vi "niRFUtil WFM Replace Waveform Segment (real wfm).vi"(4 "Waveform Segment":T2 {"y" min=0 max=127 format="%.2f"; "dx" format="%^.2e"; "x0" format="%^.2e"}, 5 "WFM replace mode":T1, 6 "Default Value (0)":sgl min=0 max=127 format="%.2f", 7 "Waveform In":T2 {"y" min=0 max=127 format="%.2f"; "dx" format="%^.2e"; "x0" format="%^.2e"}) -> (3 "Waveform Out":T2 {"y" min=0 max=127 format="%.2f"; "dx" format="%^.2e"; "x0" format="%^.2e"})   [LabVIEW 2015, in "niRFUtil.lvlib"]
doc: "(c) Copyright 2006, National Instruments, Inc. This VI may not be duplicated, sold, or distributed without written consent from National Instruments."
uses:
  niRFUtil.lvlib
  Includes/niRFUtil INC Real Waveform.ctl
  Includes/niRFUtil INC Real Array.ctl
  Includes/niRFUtil INC Waveform Replace Mode.ctl
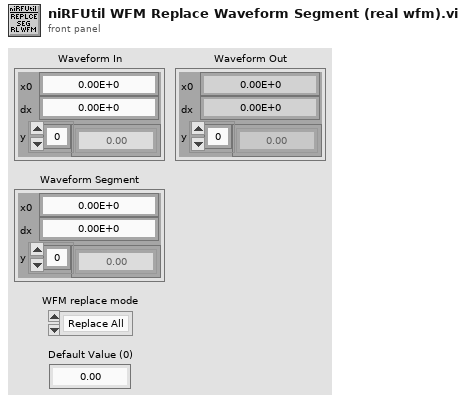
[diagram p1: front panel]
types:
  T1 = typedef "niRFUtil.lvlib/niRFUtil INC Waveform Replace Mode.ctl" = enum16{"Replace All", "Replace Pt By Pt"}
  T2 = typedef "niRFUtil.lvlib/niRFUtil INC Real Waveform.ctl" = cluster{"x0":dbl, "dx":dbl, "y":T3}
  T3 = typedef "niRFUtil.lvlib/niRFUtil INC Real Array.ctl" = sgl[]
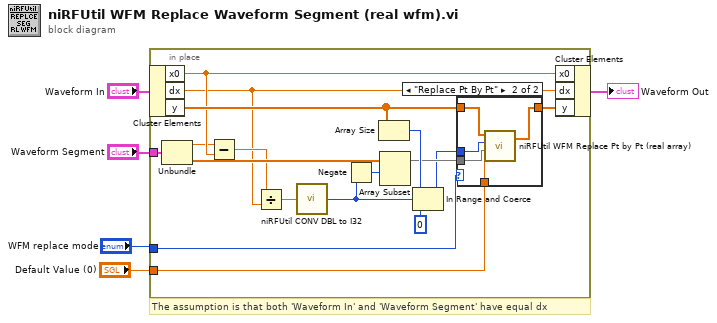
[diagram p0: block diagram]
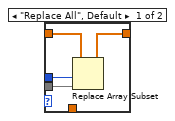
[diagram p2: hidden frame]
diagram:
  # "The assumption is that both 'Waveform In' and 'Waveform Segment' have equal dx"
  n1 = in-place {
    in-place-border: "Waveform Segment" -> [w22]
    in-place-border: "WFM replace mode" -> [w13]
    in-place-border: "Default Value (0)" -> [w12]
    n2 = in-place-cluster #1("Waveform In") -> ("x0"=w9:dbl, "dx"=w7:dbl, "y"=w15:T3)
    n3 = Unbundle(w22) -> ("x0"=w8:dbl, "y"=w19:T3)  [unwired: 1 out]
    n4 = Subtract(x=w8, y=w9) -> (x-y=w11:dbl)
    n5 = Divide(x=w11, y=w7) -> (x/y=w10:dbl)
    n6 = call "niRFUtil CONV DBL to I32.vi"("Numeric (DBL)"=w10) -> ("Numeric (I32)"=w6:i32)  [unwired: 14 in]
    n7 = Negate(x=w6) -> (-x=w16:i32)
    n8 = Array Size(array=w15) -> (size(s)=w20:i32)
    n9 = Array Subset(array=w19, index=w16) -> (w18:T3)  [unwired: 1 in]
    n10 = In Range and Coerce(upper limit=w20, x=w6, lower limit=0) -> (coerced(x)=w17:i32)  [unwired: 1 out]
    n11 = case shown="\"Replace Pt By Pt\"" w13 {
      tunnel: w18 -> [w26 w30]
      tunnel: w17 -> [w25 w29]
      tunnel: w15 -> [w24 w31]
      tunnel: [w23 w28] -> w14
      tunnel: w12 -> [_ w27]
      frame "Replace All", Default {
        n12 = Replace Array Subset(array=w24, new element=w26, index=w25) -> (w23:T3)
      }
      frame "Replace Pt By Pt" {
        n13 = call "niRFUtil WFM Replace Pt by Pt (real array).vi"("Real Array In"=w31, "Replace Index"=w29, "Replace With"=w30, "Default Value (0)"=w27) -> ("Real Array Out"=w28:T3)  [unwired: 2 in]
      }
    }
    n14 = in-place-cluster #1("x0"=w9, "dx"=w7, "y"=w14) -> (→"Waveform Out":T2)
  }
